vi "Manual IV_K237_K6485_V1.4 with XML Output.vi"() -> ()   [LabVIEW 2009]
uses:
  <vilib>/xml/Close Reference(Node).vi
  IT_Cycle_K237_K6485/subVIs/Kei237/KE237.LLB/Keith 237 Operate/Standby.vi
  <vilib>/Utility/file.llb/Write To Spreadsheet File (string).vi
  <vilib>/Utility/file.llb/Write To Spreadsheet File (DBL).vi
  <vilib>/xml/NI_XML.lvlib
panel:
  in  "Stop Loop":bool=TRUE
  out "error out 5":T1
  in  "Emergency Stop":bool
  in  "Absolute?":bool
  out "Bias":dbl
  in  "Bias Loop":bool
  out "error out 4":T1
  in  "Set Voltage Start":dbl
  in  "Set Lower Voltage Limit":dbl=-1.0
  in  "Device ID":string
  out "Running?":bool
  in  "Halt Program":bool
  in  "error in (no error)":errorcluster
  out "error out 3":errorcluster
  out "error out 2":errorcluster
  out "6485 BOTTOM (GPIB 14)":cluster{"Y":dbl[], "Y":dbl[]}[](graph)
  out "6485 TOP (GPIB 10)":cluster{"Y":dbl[], "Y":dbl[]}[](graph)
  out "237 Current (GPIB 16)":cluster{"Y":dbl[], "Y":dbl[]}[](graph) caption="Total Current"
  in  "Set Upper Voltage Limit":dbl=10.0
  in  "Voltage Steps":dbl=1.0
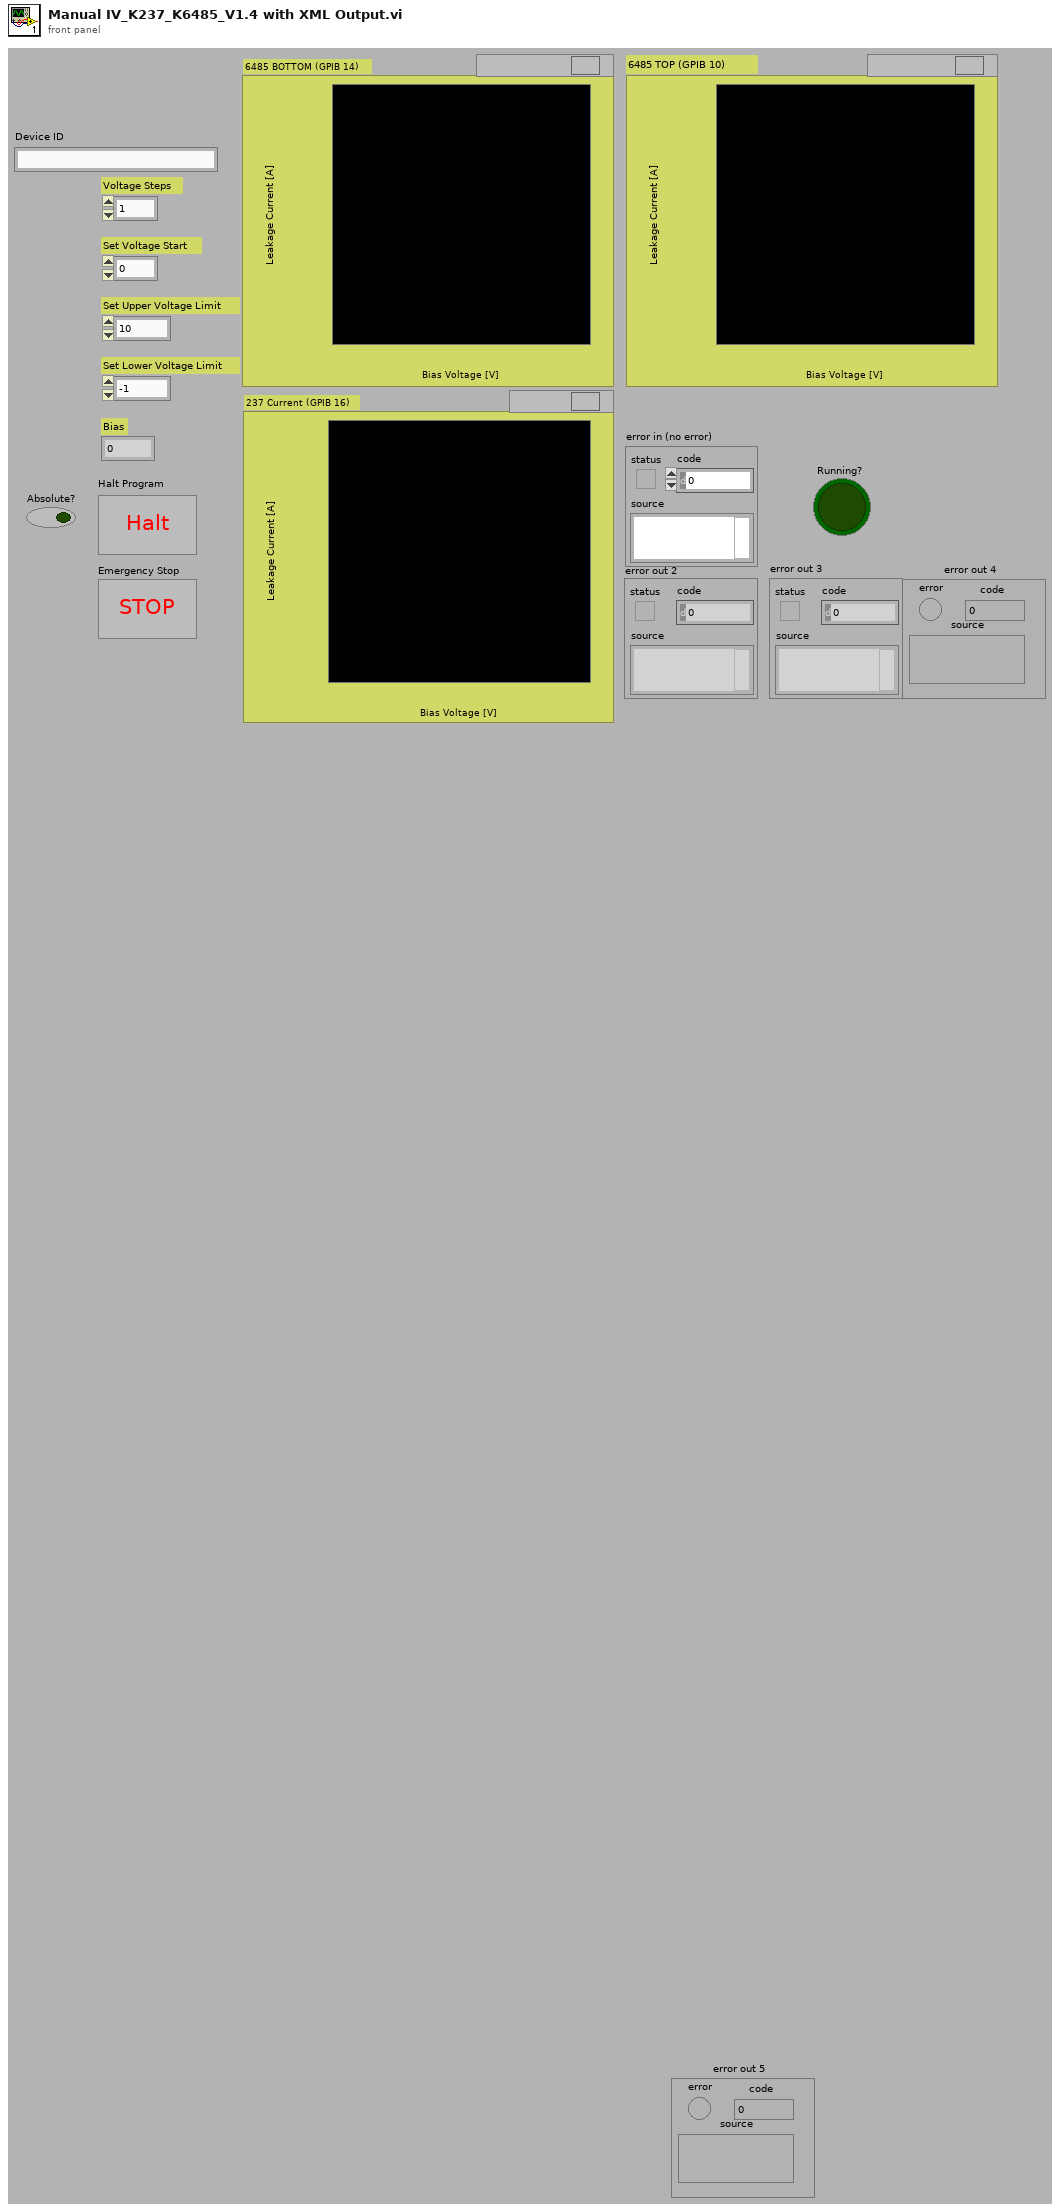
[diagram p1: front panel]
types:
  T1 = cluster{"error":bool, "code":i32, "source":string}
  T2 = enum16{"open", "replace", "create", "open or create", "replace or create", "replace or create with confirmation"}
  T3 = cluster{"Comment":string, "Part Name":string, "Kind of Part":string, "User":string}
  T4 = typedef "Semaphore RefNum" = refnum<k1>
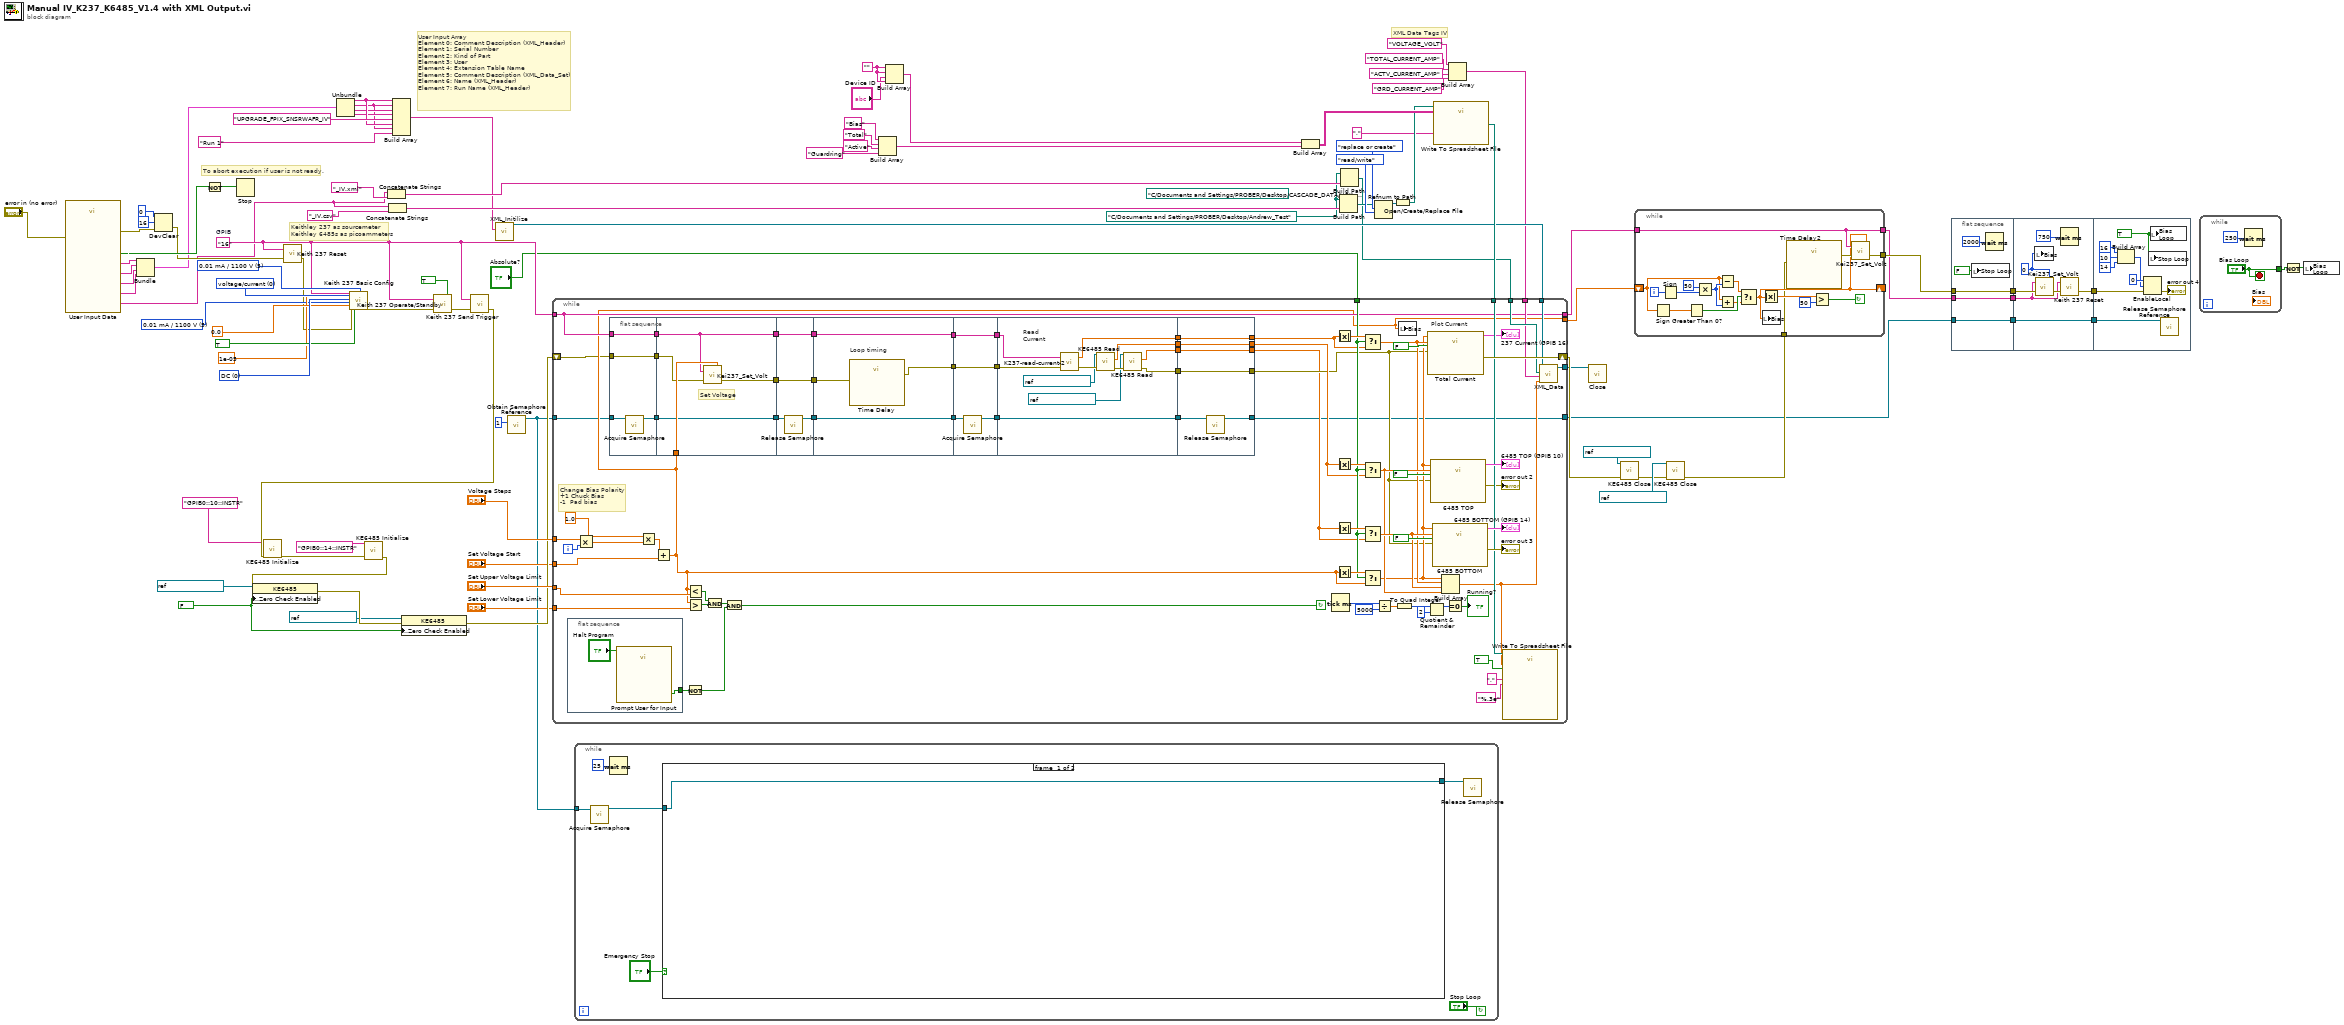
[diagram p0: block diagram]
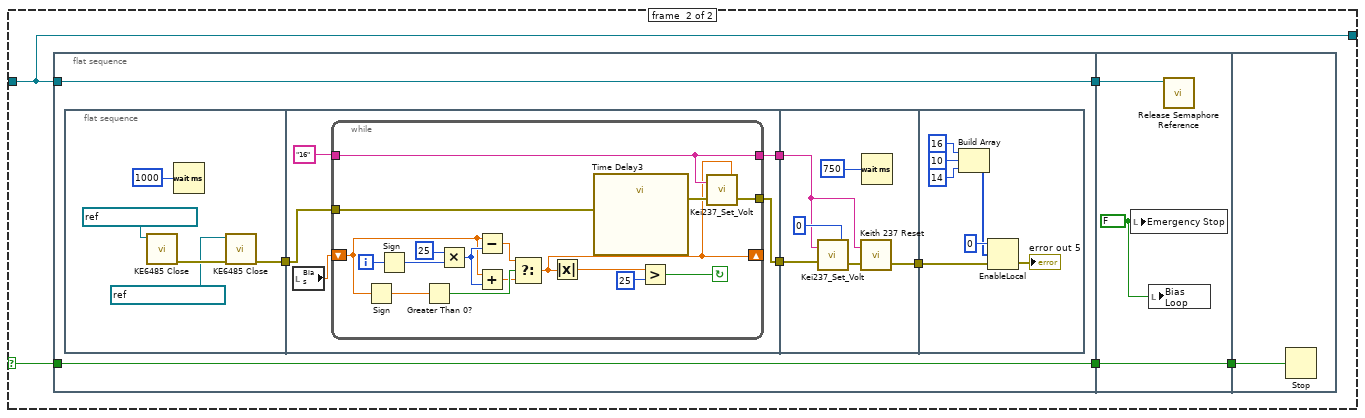
[diagram p2: hidden frame]
diagram:
  w38 = path "C:/Documents and Settings/PROBER/Desktop/Andrew_Test" ("base path")
  w14 = FALSE
  w70 = ""
  (unwired) path "C:/Documents and Settings/PROBER/Desktop/CASCADE_DATA/HPK_PIXEL_SENSORS_CV_IV/FZ320P_FPIX_after_irradiation/HPK_FZ320P_06_FPIX_1_after_irradiation" ("base path")
  w83 = u16 5 items=["auto / auto", "1 nA / 1.1 V", "10 nA / 11 V", "100 nA / 110 V", "0.001 mA / 1100 V", "0.01 mA / 1100 V", "0.1 mA / 1100 V", "1 mA / 1100 V", "10 mA / 1100 V", "100 mA / 1100 V"] ("source range\nI source / V source (auto:0)")
  w90 = u16 0 items=["voltage/current", "current/voltage"] ("source/measure (V/I:0)")
  w91 = u16 5 items=["auto / auto", "1 nA / 1.1 V", "10 nA / 11 V", "100 nA / 110 V", "0.001 mA / 1100 V", "0.01 mA / 1100 V", "0.1 mA / 1100 V", "1 mA / 1100 V", "10 mA / 1100 V", "100 mA / 1100 V"] ("compliance/\nmeasurement range (auto:0)")
  w94 = u16 0 items=["DC", "sweep"] ("function (DC:0)")
  w79 = "16"  # GPIB
  # "User Input Array\nElement 0: Comment Description (XML_Header)\nElement 1: Serial Number\nElement 2: Kind of Part\nElement 3: User\nElement 4: Extension Table Name\nElement 5: Comment Description (XML_Data_Set)\nElement 6: Name (XML_Header)\nElement 7: Run Name (XML_Header)"
  # "XML Data Tags IV"
  # "Keithley 237 as sourcemeter\nKeithley 6485s as picoammeters"
  # "To abort execution if user is not ready."
  n1 = call "User Input Data"("error in (no error)"="error in (no error)") -> ("User"=w9:string, "Kind of Part"=w10:string, "Part Name"=w11:string, "Comment"=w12:string, "Test Name"=w13:string, "OK"=w77:bool, "error out"=w42:errorcluster)  [unwired: 12 in]
  n2 = Bundle("Comment"=w12, "Part Name"=w11, "Kind of Part"=w10, "User"=w9) -> (w7:T3)  [unwired: 1 in]
  n3 = DevClear(2:w42, 3:16, 4:0) -> (0:w41:errorcluster)  [unwired: 1 out]
  n4 = Not(x=w77) -> (.not. x?=w76:bool)
  n5 = Stop(stop? (T)=w76) -> ()
  n6 = call "Keith 237 Reset.vi"("GPIB address"=w79, "error in"=w41) -> ("error out"=w78:T1)
  n7 = Unbundle(w7) -> ("Comment"=w5:string, "Part Name"=w2:string, "Kind of Part"=w3:string, "User"=w4:string)
  n8 = call "Keith 237 Basic Config.vi"("GPIB address"=w79, "source/measure (V/I:0)"=w90, "function (DC:0)"=w94, "source range\nI source / V source (auto:0)"=w83, "source level"=0.0, "error in"=w78, "1100 V range (disabled:F)"=TRUE, "current \ncompliance level"=1e-05 ("voltage \ncompliance level"), "compliance/\nmeasurement range (auto:0)"=w91) -> ("error out"=w25:T1)  [unwired: 7 in, 3 out]
  n9 = Concatenate Strings(w13, "_IV.xml" ("string")) -> (w53:string)
  n10 = Concatenate Strings(w13, "_IV.csv" ("string")) -> (w80:string)
  n11 = Build Array(w5, w2, w3, w4, "UPGRADE_FPIX_SNSRWAFR_IV", w5, w2, "Run 1" ("element")) -> (w8:string[])
  n12 = call "Keith 237 Operate/Standby.vi"("source"=TRUE, "error in"=w25, "GPIB address"=w79) -> ("error out"=w95:T1)
  n13 = call "Keith 237 Send Trigger.vi"("GPIB address"=w79, "error in"=w95) -> ("error out"=w65:T1)
  n14 = call <instrlib>:"KE6485 Initialize.vi"("error in (no error)"=w65, "resource name"="GPIB0::10::INSTR") -> ("error out"=w63:errorcluster)  [unwired: 8 in, 1 out]
  n15 = call <instrlib>:"KE6485 Initialize.vi"("error in (no error)"=w63, "resource name"="GPIB0::14::INSTR") -> ("error out"=w60:errorcluster)  [unwired: 8 in, 1 out]
  n16 = property class="KE6485"(reference=refnum<k15> "GPIB0::10::INSTR", error in=w60, "System Settings:Zero Check Enabled"=w14) -> (error out=w59:errorcluster)  [unwired: 1 out]
  n17 = property class="KE6485"(reference=refnum<k15> "GPIB0::14::INSTR", error in=w59, "System Settings:Zero Check Enabled"=w14) -> (error out=w58:errorcluster)  [unwired: 1 out]
  n18 = call "XML_Initilize.vi"("User Input"=w8) -> ("DOM document out"=w34:refnum<k20>)  [unwired: 10 in]
  n19 = call <vilib>:"Obtain Semaphore Reference.vi"("size (1)"=1) -> ("semaphore"=w19:T4)  [unwired: 4 in, 2 out]
  n20 = while {
    tunnel: w19 -> [w99]
    stop <- "Stop Loop" continue-if-true
    n21 = call <vilib>:"Acquire Semaphore.vi"("semaphore"=w99) -> ("semaphore out"=w98:T4)  [unwired: 4 in, 2 out]
    n22 = Wait (ms)(milliseconds to wait=25) -> ()  [unwired: 1 out]
    n23 = case shown="True" "Emergency Stop" {
      selector: "Emergency Stop" -> [_ w107]
      tunnel: w98 -> [w102 w103]
      tunnel: [w102 w103] -> w97
      frame #0 {
      }
      frame #1 {
        n24 = flat-sequence {
          tunnel: [w113] -> w106
          tunnel: w107 -> [w113]
          tunnel: w103 -> [w108]
          tunnel: [w108] -> w104
          tunnel: w106 -> [w156]
          tunnel: [w156] -> w105
          tunnel: w104 -> [w154]
          tunnel: w105 -> [w157]
          frame #0 {
            n25 = flat-sequence {
              tunnel: [w114] -> w111
              tunnel: w111 -> [w120]
              tunnel: [w121] -> w110
              tunnel: [w122] -> w109
              tunnel: [w144] -> w112
              tunnel: w110 -> [w142]
              tunnel: w109 -> [w141]
              tunnel: w112 -> [w151]
              frame #0 {
                n26 = call "KE6485 Close.vi"("instrument handle"=refnum<k15> "GPIB0::10::INSTR") -> ("error out"=w117:errorcluster)  [unwired: 10 in]
                n27 = Wait (ms)(milliseconds to wait=1000) -> ()  [unwired: 1 out]
                n28 = call "KE6485 Close.vi"("error in (no error)"=w117, "instrument handle"=refnum<k15> "GPIB0::14::INSTR") -> ("error out"=w114:errorcluster)  [unwired: 9 in]
              }
              frame #1 {
                n29 = local read "Bias"() -> (w119:dbl)
                n30 = while {
                  tunnel: [w140] -> w121
                  tunnel: "16" ("GPIB") -> [w136]
                  tunnel: [w136] -> w122
                  shift-right: [w125] -> _
                  shift-left: w119 -> [w131]
                  tunnel: w120 -> [w124]
                  i -> [w127]
                  stop <- w128 continue-if-true
                  n31 = Sign(1:w131) -> (0:w129:dbl)
                  n32 = Sign(1:w127) -> (0:w126:i32)
                  n33 = Greater Than 0?(x=w129) -> (x > 0?=w135:bool)
                  n34 = Multiply(x=25, y=w126) -> (x*y=w134:i32)
                  n35 = Subtract(x=w131, y=w134) -> (x-y=w133:dbl)
                  n36 = Add(x=w131, y=w134) -> (x+y=w132:dbl)
                  n37 = Select(t=w133, s=w135, f=w132) -> (s? t:f=w125:dbl)
                  n38 = Absolute Value(x=w125) -> (abs(x)=w130:dbl)
                  n39 = call "Time Delay3"("error in (no error)"=w124) -> ("error out"=w137:errorcluster)  [unwired: 10 in]
                  n40 = Greater?(x=w130, y=25) -> (0:w128:bool)
                  n41 = call "Kei237_Set_Volt.vi"("Voltage"=w125, "error in"=w137, "GPIB"=w136) -> ("error out"=w140:errorcluster)
                }
              }
              frame #2 {
                n42 = call "Kei237_Set_Volt.vi"("Voltage"=0, "error in"=w142, "GPIB"=w141) -> ("error out"=w146:errorcluster)
                n43 = call "Keith 237 Reset.vi"("GPIB address"=w141, "error in"=w146) -> ("error out"=w144:T1)
                n44 = Wait (ms)(milliseconds to wait=750) -> ()  [unwired: 1 out]
              }
              frame #3 {
                n45 = Build Array(16, 10, 14) -> (w147:i32[])
                n46 = EnableLocal(2:w151, 3:w147, 4:0) -> (0:→"error out 5":errorcluster)  [unwired: 1 out]
              }
            }
          }
          frame #1 {
            w155 = FALSE ("Emergency Stop")
            n47 = local write "Emergency Stop"(w155) -> ()
            n48 = local write "Bias Loop"(w155) -> ()
            n49 = call <vilib>:"Release Semaphore Reference.vi"("semaphore"=w154) -> ()  [unwired: 9 in, 2 out]
          }
          frame #2 {
            n50 = Stop(stop? (T)=w157) -> ()
          }
        }
      }
    }
    n51 = call <vilib>:"Release Semaphore.vi"("semaphore"=w97) -> ()  [unwired: 5 in, 2 out]
  }
  n52 = Build Array("Bias", "Total", "Active", "Guardring") -> (w68:string[])
  n53 = Build Array(w70, w70, "Device ID", w70) -> (w69:string[])
  n54 = Build Array(w69, w68) -> (w75:string[][])
  n55 = Build Path(base path=w38, name or relative path=w80) -> (appended path=w67:path)
  n56 = Build Path(base path=w38, name or relative path=w53) -> (appended path=w33:path)
  n57 = Open/Create/Replace File(file path (use dialog)=w67, operation (0:open)=T2."replace or create", access (0:read/write)=enum16{"read/write", "read-only", "write-only"}."read/write") -> (refnum out=w56:refnum<file>)  [unwired: 1 in, 4 out]
  n58 = Refnum to Path(1:w56) -> (0:w55:path)
  n59 = call-poly <vilib>:"Write To Spreadsheet File.vi"("delimiter (\\t)"="," ("file format"), "2D data"=w75, "file path (dialog if empty)"=w55) -> ("new file path (Not A Path if cancelled)"=w54:path)  [unwired: 5 in]
  n60 = Build Array("VOLTAGE_VOLT", "TOTAL_CURRENT_AMP", "ACTV_CURRENT_AMP", "GRD_CURRENT_AMP") -> (w28:string[])
  n61 = while {
    tunnel: w79 -> [w187]
    tunnel: "Set Upper Voltage Limit" -> [w233]
    tunnel: "Voltage Steps" -> [w232]
    tunnel: [w187] -> w47
    shift-right: [w225] -> w48
    shift-left: w58 -> [w185]
    tunnel: w54 -> [w224]
    tunnel: "Set Lower Voltage Limit" -> [w211]
    tunnel: "Set Voltage Start" -> [w209]
    tunnel: [w186] -> w45
    tunnel: w34 -> [w203]
    tunnel: w33 -> [w202]
    tunnel: w28 -> [w201]
    tunnel: [w200] -> w27
    tunnel: "Absolute?" -> [w189]
    tunnel: w19 -> [w165]
    tunnel: [w158] -> w18
    i -> [w234]
    stop <- w176 continue-if-true
    # "Change Bias Polarity\n+1 Chuck Bias\n-1  Pad bias"
    # "Plot Current"
    n62 = flat-sequence {
      tunnel: [w235] -> w204
      frame #0 {
        n63 = call "Prompt User for Input"("Enable"="Halt Program") -> ("Yes"=w235:bool)  [unwired: 17 in, 1 out]
      }
    }
    n64 = Multiply(x=w232, y=w234) -> (x*y=w215:dbl)
    n65 = flat-sequence {
      tunnel: w185 -> [w239]
      tunnel: w187 -> [w240]
      tunnel: [w240] -> w175
      tunnel: [w239] -> w174
      tunnel: w165 -> [w238]
      tunnel: [w237] -> w163
      tunnel: [w241] -> w173
      tunnel: w186 -> [w245]
      tunnel: [w243] -> w171
      tunnel: w175 -> [w241]
      tunnel: w174 -> [w244]
      tunnel: [w242] -> w164
      tunnel: w163 -> [w242]
      tunnel: w173 -> [w249]
      tunnel: [w249] -> w172
      tunnel: w171 -> [w248]
      tunnel: [w248] -> w170
      tunnel: w164 -> [w247]
      tunnel: [w246] -> w161
      tunnel: w172 -> [w252]
      tunnel: w170 -> [w251]
      tunnel: [w253] -> w169
      tunnel: [w252] -> w167
      tunnel: [w250] -> w162
      tunnel: w161 -> [w250]
      tunnel: w169 -> [w257]
      tunnel: [w257] -> w168
      tunnel: w167 -> [w256]
      tunnel: [w256] -> w166
      tunnel: w162 -> [w255]
      tunnel: [w254] -> w159
      tunnel: w168 -> [w268]
      tunnel: w166 -> [w267]
      tunnel: [w264] -> w180
      tunnel: [w266] -> w179
      tunnel: [w265] -> w178
      tunnel: [w263] -> w177
      tunnel: [w258] -> w160
      tunnel: w159 -> [w258]
      tunnel: [w271] -> w181
      tunnel: [w272] -> w183
      tunnel: [w273] -> w184
      tunnel: [w274] -> w182
      tunnel: w180 -> [w274]
      tunnel: w179 -> [w273]
      tunnel: w178 -> [w272]
      tunnel: w177 -> [w271]
      tunnel: w160 -> [w270]
      tunnel: [w269] -> w158
      frame #0 {
        n66 = call <vilib>:"Acquire Semaphore.vi"("semaphore"=w238) -> ("semaphore out"=w237:T4)  [unwired: 4 in, 2 out]
      }
      frame #1 {
        # "Set Voltage"
        n67 = call "Kei237_Set_Volt.vi"("Voltage"=w245, "error in"=w244, "GPIB"=w241) -> ("error out"=w243:errorcluster)
      }
      frame #2 {
        n68 = call <vilib>:"Release Semaphore.vi"("semaphore"=w247) -> ("semaphore out"=w246:T4)  [unwired: 5 in, 1 out]
      }
      frame #3 {
        # "Loop timing"
        n69 = call "Time Delay"("error in (no error)"=w251) -> ("error out"=w253:errorcluster)  [unwired: 10 in]
      }
      frame #4 {
        n70 = call <vilib>:"Acquire Semaphore.vi"("semaphore"=w255) -> ("semaphore out"=w254:T4)  [unwired: 4 in, 2 out]
      }
      frame #5 {
        # "Read \nCurrent"
        n71 = call "K237-read-current-2.vi"("error in"=w268, "GPIB"=w267) -> ("error out"=w262:T1, "Current"=w266:dbl)
        n72 = call <instrlib>:"KE6485 Read.vi"("error in (no error)"=w262, "instrument handle"=refnum<k15> "GPIB0::10::INSTR") -> ("error out"=w260:errorcluster, "reading"=w265:dbl)  [unwired: 7 in, 1 out]
        n73 = call <instrlib>:"KE6485 Read.vi"("error in (no error)"=w260, "instrument handle"=refnum<k15> "GPIB0::14::INSTR") -> ("error out"=w264:errorcluster, "reading"=w263:dbl)  [unwired: 7 in, 1 out]
      }
      frame #6 {
        n74 = call <vilib>:"Release Semaphore.vi"("semaphore"=w270) -> ("semaphore out"=w269:T4)  [unwired: 5 in, 1 out]
      }
    }
    n75 = Multiply(x=1.0, y=w215) -> (x*y=w210:dbl)
    n76 = Add(x=w210, y=w209) -> (x+y=w186:dbl)
    n77 = Not(x=w204) -> (.not. x?=w198:bool)
    n78 = Less?(x=w186, y=w233) -> (x < y?=w208:bool)
    n79 = Greater?(x=w186, y=w211) -> (0:w207:bool)
    n80 = And(x=w208, y=w207) -> (x .and. y?=w205:bool)
    n81 = And(x=w205, y=w198) -> (x .and. y?=w176:bool)
    n82 = Tick Count (ms)() -> (millisecond timer value=w220:u32)
    n83 = Absolute Value(x=w184) -> (abs(x)=w194:dbl)
    n84 = Absolute Value(x=w183) -> (abs(x)=w195:dbl)
    n85 = Absolute Value(x=w181) -> (abs(x)=w196:dbl)
    n86 = Absolute Value(x=w186) -> (abs(x)=w197:dbl)
    n87 = Select(t=w194, s=w189, f=w184) -> (s? t:f=w191:dbl)
    n88 = Select(t=w195, s=w189, f=w183) -> (s? t:f=w192:dbl)
    n89 = Select(t=w196, s=w189, f=w181) -> (s? t:f=w193:dbl)
    n90 = Select(t=w197, s=w189, f=w186) -> (s? t:f=w190:dbl)
    n91 = Divide(x=w220, y=5000) -> (x/y=w218:dbl)
    n92 = To Quad Integer(1:w218) -> (0:w217:i64)
    n93 = local write "Bias"(w186) -> ()
    n94 = call "Total Current"("error in (no error)"=w182, "Reset"=FALSE, "Y Input"=w191, "X Input"=w190) -> ("error out"=w225:errorcluster, "XY Graph"=→"237 Current (GPIB 16)":cluster{"Y":dbl[], "Y":dbl[]}[])  [unwired: 1 in, 5 out]
    n95 = Quotient & Remainder(x=w217, y=2) -> (x-y*floor(x/y)=w221:i64)  [unwired: 1 out]
    n96 = call "6485 TOP"("error in (no error)"=w182, "Reset"=FALSE, "Y Input"=w192, "X Input"=w190) -> ("error out"=→"error out 2":errorcluster, "XY Graph"=→"6485 TOP (GPIB 10)":cluster{"Y":dbl[], "Y":dbl[]}[])  [unwired: 1 in, 5 out]
    n97 = call "6485 BOTTOM"("error in (no error)"=w182, "Reset"=FALSE, "Y Input"=w193, "X Input"=w190) -> ("error out"=→"error out 3":errorcluster, "XY Graph"=→"6485 BOTTOM (GPIB 14)":cluster{"Y":dbl[], "Y":dbl[]}[])  [unwired: 1 in, 5 out]
    n98 = Build Array(w190, w191, w193, w192) -> (w199:dbl[])
    n99 = Equal To 0?(x=w221) -> (x = 0?=→"Running?":bool)
    n100 = call-poly <vilib>:"Write To Spreadsheet File.vi"("delimiter (\\t)"="," ("file format"), "format (%.3f)"="%.3e" ("file format"), "append to file? (new file:F)"=TRUE, "1D data"=w199, "file path (dialog if empty)"=w224) -> ()  [unwired: 2 in, 2 out]
    n101 = call "XML_Data.vi"("Data Input Array"=w199, "Data Tag Names Array"=w201, "XML File Path"=w202, "DOM document in"=w203) -> ("DOM document out"=w200:refnum<k20>)  [unwired: 6 in, 1 out]
  }
  n102 = call-poly <vilib>:"Close.vi"("node"=w27) -> ()  [unwired: 8 in, 1 out]
  n103 = call "KE6485 Close.vi"("error in (no error)"=w48, "instrument handle"=refnum<k15> "GPIB0::10::INSTR") -> ("error out"=w22:errorcluster)  [unwired: 9 in]
  n104 = call "KE6485 Close.vi"("error in (no error)"=w22, "instrument handle"=refnum<k15> "GPIB0::14::INSTR") -> ("error out"=w21:errorcluster)  [unwired: 9 in]
  n105 = while {
    tunnel: [w291] -> w49
    tunnel: w47 -> [w287]
    tunnel: [w287] -> w46
    shift-right: [w276] -> _
    shift-left: w45 -> [w282]
    tunnel: w21 -> [w275]
    i -> [w278]
    stop <- w279 continue-if-true
    n106 = Sign(1:w282) -> (0:w280:dbl)
    n107 = Sign(1:w278) -> (0:w277:i32)
    n108 = Greater Than 0?(x=w280) -> (x > 0?=w286:bool)
    n109 = Multiply(x=50, y=w277) -> (x*y=w285:i32)
    n110 = Subtract(x=w282, y=w285) -> (x-y=w284:dbl)
    n111 = Add(x=w282, y=w285) -> (x+y=w283:dbl)
    n112 = Select(t=w284, s=w286, f=w283) -> (s? t:f=w276:dbl)
    n113 = Absolute Value(x=w276) -> (abs(x)=w281:dbl)
    n114 = local write "Bias"(w276) -> ()
    n115 = call "Time Delay2"("error in (no error)"=w275) -> ("error out"=w288:errorcluster)  [unwired: 10 in]
    n116 = Greater?(x=w281, y=50) -> (0:w279:bool)
    n117 = call "Kei237_Set_Volt.vi"("Voltage"=w276, "error in"=w288, "GPIB"=w287) -> ("error out"=w291:errorcluster)
  }
  n118 = flat-sequence {
    tunnel: w46 -> [w295]
    tunnel: w49 -> [w296]
    tunnel: [w296] -> w44
    tunnel: [w295] -> w43
    tunnel: w18 -> [w292]
    tunnel: [w292] -> w16
    tunnel: w44 -> [w302]
    tunnel: w43 -> [w301]
    tunnel: [w299] -> w37
    tunnel: [w297] -> w17
    tunnel: w16 -> [w297]
    tunnel: w37 -> [w310]
    tunnel: w17 -> [w308]
    frame #0 {
      n119 = local write "Stop Loop"(FALSE ("Stop Loop")) -> ()
      n120 = Wait (ms)(milliseconds to wait=2000) -> ()  [unwired: 1 out]
    }
    frame #1 {
      w300 = 0
      n121 = local write "Bias"(w300) -> ()
      n122 = call "Kei237_Set_Volt.vi"("Voltage"=w300, "error in"=w302, "GPIB"=w301) -> ("error out"=w303:errorcluster)
      n123 = call "Keith 237 Reset.vi"("GPIB address"=w301, "error in"=w303) -> ("error out"=w299:T1)
      n124 = Wait (ms)(milliseconds to wait=750) -> ()  [unwired: 1 out]
    }
    frame #2 {
      w309 = TRUE ("Bias Loop")
      n125 = Build Array(16, 10, 14) -> (w304:i32[])
      n126 = EnableLocal(2:w310, 3:w304, 4:0) -> (0:→"error out 4":errorcluster)  [unwired: 1 out]
      n127 = local write "Stop Loop"(w309) -> ()
      n128 = local write "Bias Loop"(w309) -> ()
      n129 = call <vilib>:"Release Semaphore Reference.vi"("semaphore"=w308) -> ()  [unwired: 9 in, 2 out]
    }
  }
  n130 = while {
    tunnel: ["Bias Loop"] -> w36
    stop <- "Bias Loop" stop-if-true
    n131 = Wait (ms)(milliseconds to wait=250) -> ()  [unwired: 1 out]
  }
  n132 = Not(x=w36) -> (.not. x?=w35:bool)
  n133 = local write "Bias Loop"(w35) -> ()
